vi "SECoP-putCommandAnswer.vi"(5 "sigma (SECoP_data)":T1 {"ptr64" format="%.0x"; "ptr32" format="%.0x"}, 6 "timestamp":dbl=nan, 7 "command id":u64, 8 "error in (no error)":errorcluster, 9 "value (SECoP_data)":T1 {"ptr64" format="%.0x"; "ptr32" format="%.0x"}, 10 "SECoP error":T2 items=["warn: missing properties"=4, "warn: buffer too small"=3, "warn: custom property"=2, "warn: no description"=1, "success"=0, "error: unknown command"=-1, "error: invalid name"=-2, "error: invalid node"=-3, "error: invalid module"=-4, "error: invalid parameter"=-5, "error: invalid property"=-6, "error: invalid command"=-7, "error: not implemented"=-8, "error: readonly"=-9, "error: no data"=-10, "error: no memory"=-11, "error: not initialized"=-12, "error: invalid value"=-13, "error: missing mandatory prop"=-14, "error: no setter/getter"=-15, "error: no setter"=-16, "error: no getter"=-17, "error: name already in use"=-18], 11 "DLL path (in)":T3) -> (0 "error out":errorcluster, 3 "DLL path (out)":T3)   [LabVIEW 2023, in "SECoP.lvlib"]
doc: "Call <b>\"SECoP-putCommandAnswer.vi\"</b>, when \"SECoP-getStoredCommand.vi\" or \"SECoP-filterStoredCommand.vi\" provided a to do action. You have to provide the read value, value after change or command call result. All clients which subscribed to this module should be informed about parameter values.\n\nYour have to call this VI after a successful result from functions before. If your handling was successful, provide a \"success\" error code for this VI. If you encounter an error while handling the action, e.g. communication problem with your device, you should provide a meaningful error code.\n\n<b>DLL path</b> input and output of cluster from \"SECoP-Initialize.vi\"\n<b>command id</b> command id from \"SECoP-getStoredCommand.vi\" or \"SECoP-filterStoredCommand.vi\"\n<b>SECoP error</b> result of the action\n<b>value (SECoP_data)</b> actual/new value of parameter, result of \"do\"-command call\n<b>sigma (SECoP_data)</b> if applicable, the error bar of the actual/new value of parameter\n<b>timestamp</b> time in seconds (with fraction) from 1970/1/1 0:0am of data (or NaN for actual time)"
uses:
  SECoP.lvlib
  SECoP-libraries.ctl
  SECoP-error.ctl
  SECoP-data/SECoP-data.ctl
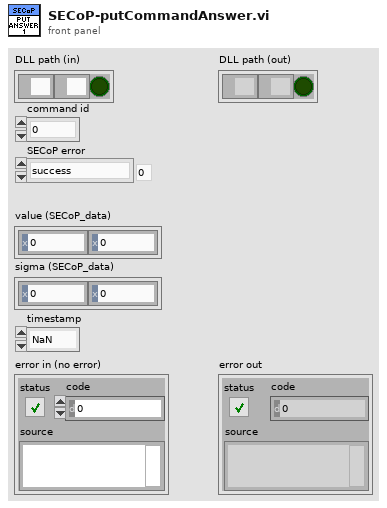
[diagram p1: front panel]
types:
  T1 = typedef "SECoP.lvlib/SECoP-data.ctl" = cluster{"ptr32":u32, "ptr64":u64}
  T2 = typedef "SECoP.lvlib/SECoP-error.ctl" = i32
  T3 = typedef "SECoP.lvlib/SECoP-libraries.ctl" = cluster{"serverDLL":path, "variantDLL":path, "cleanup_mode":bool}
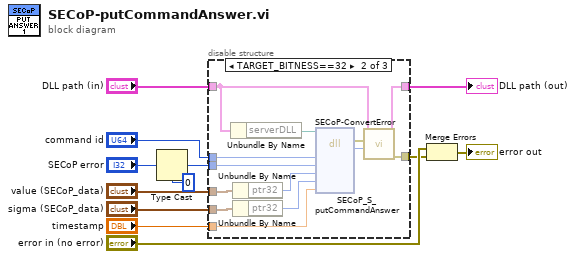
[diagram p0: block diagram]
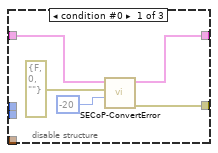
[diagram p2: hidden frame]
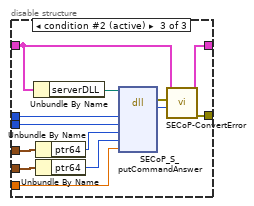
[diagram p3: hidden frame]
diagram:
  n1 = Type Cast(type=0 ("SECoP error"), x="SECoP error") -> (*(type *) &x=w1:i32)
  n2 = disable-structure shown="TARGET_BITNESS==32" {
    disable-tunnel: [w14 w20 w32] -> w12
    disable-tunnel: "DLL path (in)" -> [w16 w21 w33]
    disable-tunnel: [w15 w18 w34] -> w5
    disable-tunnel: "command id" -> [_ w30 w41]
    disable-tunnel: w1 -> [_ w29 w42]
    disable-tunnel: "timestamp" -> [_ w28 w43]
    disable-tunnel: "value (SECoP_data)" -> [_ w27 w40]
    disable-tunnel: "sigma (SECoP_data)" -> [_ w25 w37]
    frame condition #0 {
      n3 = call "SECoP-ConvertError.vi"("return code"=-20, "error in (no error)"=errorcluster {"status"=FALSE, "code"=0, "source"=""}, "DLL path (in)"=w16) -> ("error out"=w15:errorcluster, "DLL path (out)"=w14:T3)  [unwired: 7 in]
    }
    frame condition #1 {
      n4 = Unbundle By Name(w21) -> ("serverDLL"=w23:path)
      n5 = Unbundle By Name(w27) -> ("ptr32"=w26:u32)
      n6 = Unbundle By Name(w25) -> ("ptr32"=w24:u32)
      n7 = dll-call lib="Z:/Praktische Aufgaben/SECoP-LabVIEW2015/32bit/SECoP32.dll" fn="SECoP_S_putCommandAnswer"(path in=w23, "id"=w30, "SECoP error"=w29, "value"=w26, "sigma"=w24, "timestamp"=w28) -> (error out=w22:errorcluster, "return type"=w19:i32)  [unwired: 7 in, 1 out]
      n8 = call "SECoP-ConvertError.vi"("return code"=w19, "error in (no error)"=w22, "DLL path (in)"=w21) -> ("error out"=w18:errorcluster, "DLL path (out)"=w20:T3)  [unwired: 7 in]
    }
    frame condition #2 (active) {
      n9 = Unbundle By Name(w33) -> ("serverDLL"=w38:path)
      n10 = Unbundle By Name(w40) -> ("ptr64"=w39:u64)
      n11 = Unbundle By Name(w37) -> ("ptr64"=w36:u64)
      n12 = dll-call lib="Z:/Praktische Aufgaben/SECoP-LabVIEW2015/32bit/SECoP32.dll" fn="SECoP_S_putCommandAnswer"(path in=w38, "id"=w41, "SECoP error"=w42, "value"=w39, "sigma"=w36, "timestamp"=w43) -> (error out=w35:errorcluster, "return type"=w31:i32)  [unwired: 7 in, 1 out]
      n13 = call "SECoP-ConvertError.vi"("return code"=w31, "error in (no error)"=w35, "DLL path (in)"=w33) -> ("error out"=w34:errorcluster, "DLL path (out)"=w32:T3)  [unwired: 7 in]
    }
  }
  "DLL path (out)" <- w12
  n14 = Merge Errors("error in (no error)", w5) -> (→"error out":errorcluster)
